vi "Calcolo SCORRIMENTO.vi"(7 "POLI":u16, 9 "FREQ":dbl, 10 "RPM":dbl) -> (2 "SCORRIMENTO":dbl)   [LabVIEW 2019]
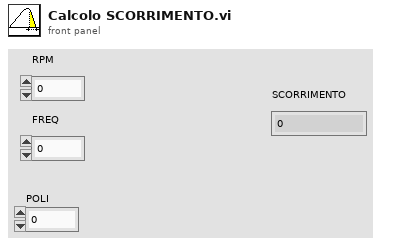
[diagram p1: front panel]
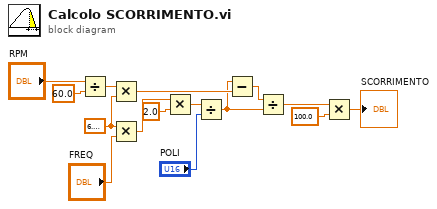
[diagram p0: block diagram]
diagram:
  w7 = 6.283185307179586
  n1 = Divide(x="RPM", y=60.0) -> (x/y=w8:dbl)
  n2 = Multiply(x=w8, y=w7) -> (x*y=w6:dbl)
  n3 = Multiply(x=w7, y="FREQ") -> (x*y=w5:dbl)
  n4 = Multiply(x=w5, y=2.0) -> (x*y=w3:dbl)
  n5 = Divide(x=w3, y="POLI") -> (x/y=w1:dbl)
  n6 = Subtract(x=w1, y=w6) -> (x-y=w13:dbl)
  n7 = Divide(x=w13, y=w1) -> (x/y=w14:dbl)
  n8 = Multiply(x=w14, y=100.0) -> (x*y=→"SCORRIMENTO":dbl)
